vi "Set Refnum.vi"(8 "error in (no error)":errorcluster, 10 "Ctl Refnum":refnum<vi>, 11 "Ctrl Refnum Value Source in":refnum<class "Ctrl Refnum Value Source.lvclass">) -> (0 "error out":errorcluster, 3 "Ctrl Refnum Value Source out":refnum<class "Ctrl Refnum Value Source.lvclass">)   [LabVIEW 2020, in "Composed Columns.lvlib" / "Ctrl Refnum Value Source.lvclass"]
uses:
  Ctrl Refnum Value Source.lvclass
  Ctrl Refnum Value Source.lvclass/Ctrl Refnum Value Source.ctl
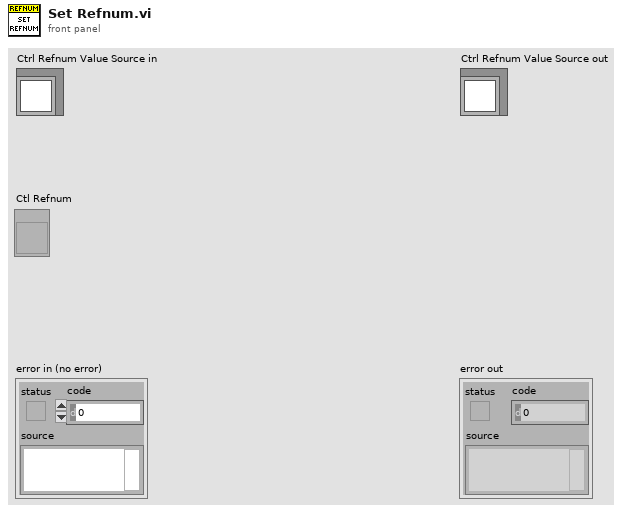
[diagram p1: front panel]
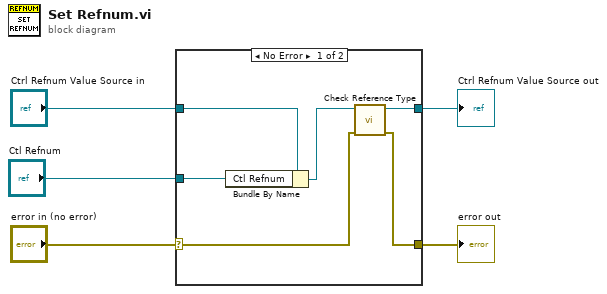
[diagram p0: block diagram]
diagram:
  n1 = case shown="No Error" "error in (no error)" {
    selector: "error in (no error)" -> [w7 w13]
    tunnel: [w6 w13] -> w4
    tunnel: [w8 w12] -> w2
    tunnel: "Ctrl Refnum Value Source in" -> [w11 w12]
    tunnel: "Ctl Refnum" -> [w10 _]
    frame No Error {
      n2 = Bundle By Name(cluster=w11, "Ctl Refnum"=w10) -> (w9:refnum<class "Ctrl Refnum Value Source.lvclass">)
      n3 = call-dynamic "Check Reference Type.vi"("error in (no error)"=w7, "Refnum Value Source in"=w9) -> ("error out"=w6:errorcluster, "Refnum Value Source out"=w8:refnum<class "Ctrl Refnum Value Source.lvclass">)  [unwired: 8 in]
    }
    frame Error {
    }
  }
  "error out" <- w4
  "Ctrl Refnum Value Source out" <- w2
